vi "Validate Fixed Header.vi"(8 "error in (no error)":errorcluster, 11 "UNSUBACK in":refnum<class "UNSUBACK.lvclass">) -> (0 "error out":errorcluster, 1 "Valid":bool, 3 "UNSUBACK out":refnum<class "UNSUBACK.lvclass">)   [LabVIEW 2013, in "UNSUBACK.lvclass"]
uses:
  UNSUBACK.lvclass
  ControlPacket/ControlPacket.lvclass/ControlPacket.ctl
  ControlPacket/ControlPacket.lvclass
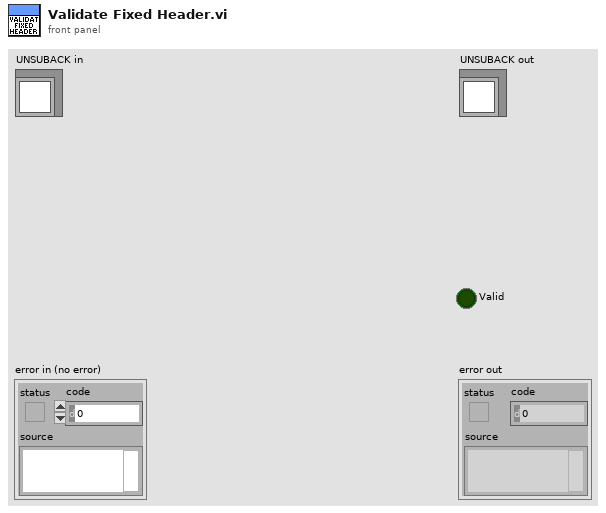
[diagram p1: front panel]
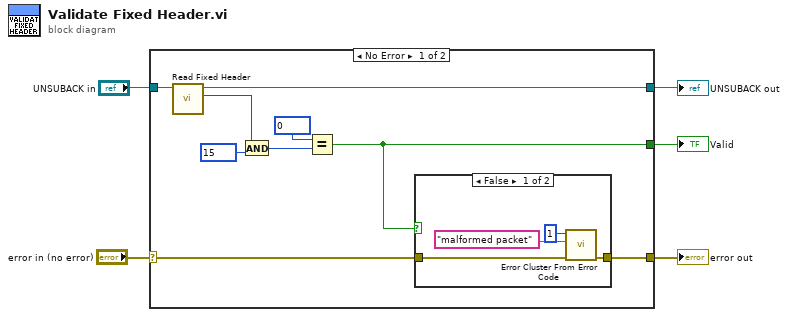
[diagram p0: block diagram]
diagram:
  n1 = case shown="No Error" "error in (no error)" {
    selector: "error in (no error)" -> [w9 w21]
    tunnel: [w8 w21] -> w3
    tunnel: [w6 _] -> w2
    tunnel: [w7 w20] -> w1
    tunnel: "UNSUBACK in" -> [w10 w20]
    frame No Error {
      n2 = call "Read Fixed Header.vi"("ControlPacket in"=w10) -> ("Fixed Header"=w13:u8, "ControlPacket out"=w7:refnum<class "UNSUBACK.lvclass">)  [unwired: 9 in]
      n3 = And(x=w13, y=u8 15) -> (x .and. y?=w12:u8)
      n4 = Equal?(x=u8 0 ("y"), y=w12) -> (x = y?=w6:bool)
      n5 = case shown="False" w6 {
        tunnel: [w16 w19] -> w8
        tunnel: w9 -> [w15 w19]
        frame False {
          n6 = call <vilib>:"Error Cluster From Error Code.vi"("error in (no error)"=w15, "error message (\"\")"="malformed packet" ("error message (\"\")"), "error code (0)"=1) -> ("error out"=w16:errorcluster)  [unwired: 6 in]
        }
        frame True {
        }
      }
    }
    frame Error {
    }
  }
  "Valid" <- w2
  "error out" <- w3
  "UNSUBACK out" <- w1
